vi "SLT Get Process Handle.vi"(0 "Process Id":i64, 11 "error in (no error)":errorcluster) -> (4 "Process handle":i64, 15 "error out":errorcluster)   [LabVIEW 2013, in "ProcessInfo.lvlib"]
doc: "Opens an existing local process object."
uses:
  ProcessInfo.lvlib
  kernel32.dll
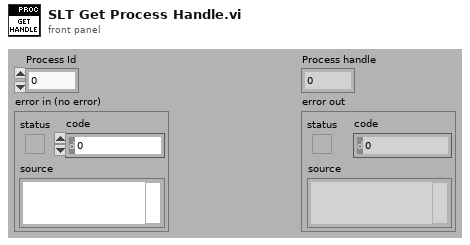
[diagram p1: front panel]
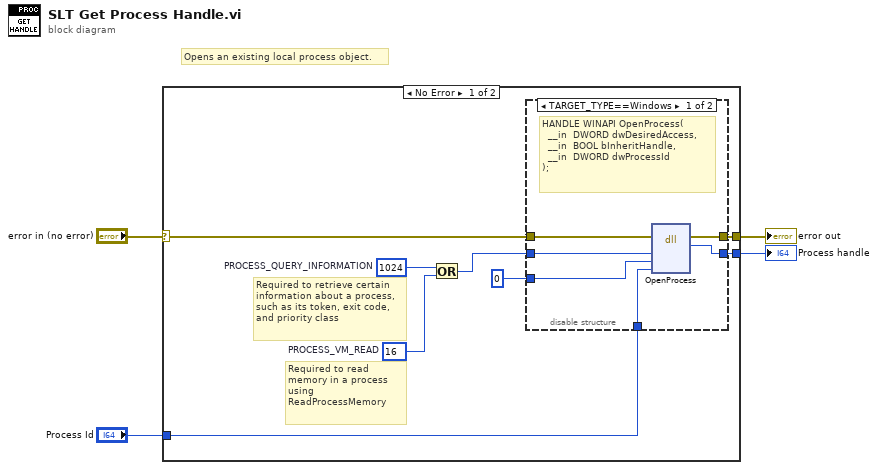
[diagram p0: block diagram]
diagram:
  # "Opens an existing local process object."
  n1 = case shown="No Error" "error in (no error)" {
    selector: "error in (no error)" -> [w5 w20]
    tunnel: [w9 _] -> w4
    tunnel: [w7 w20] -> w3
    tunnel: "Process Id" -> [w6 _]
    frame No Error {
      w12 = u32 1024  # PROCESS_QUERY_INFORMATION
      w11 = u32 16  # PROCESS_VM_READ
      # "Required to retrieve certain information about a process, such as its token, exit code, and priority class"
      # "Required to read memory in a process using ReadProcessMemory"
      n2 = Or(x=w12, y=w11) -> (x .or. y?=w10:u32)
      n3 = disable-structure shown="TARGET_TYPE==Windows" {
        disable-tunnel: w10 -> [w18 _]
        disable-tunnel: [w17 _] -> w9
        disable-tunnel: i64 0 ("InheritHandle") -> [w16 _]
        disable-tunnel: [w15 w19] -> w7
        disable-tunnel: w6 -> [w14 _]
        disable-tunnel: w5 -> [w13 w19]
        frame condition #0 (active) {
          # "HANDLE WINAPI OpenProcess(\n  __in  DWORD dwDesiredAccess,\n  __in  BOOL bInheritHandle,\n  __in  DWORD dwProcessId\n);"
          n4 = dll-call lib="kernel32.dll" fn="OpenProcess"(error in=w13, "DesiredAccess"=w18, "InheritHandle"=w16, "ProcessId"=w14) -> (error out=w15:errorcluster, "handle"=w17:i64)  [unwired: 5 in, 1 out]
        }
        frame condition #1 {
        }
      }
    }
    frame Error {
    }
  }
  "error out" <- w3
  "Process handle" <- w4
